vi "HC-Bal_Calc.vi"(7 "Omicron?":bool, 8 "HC Bal Transient":dbl, 9 "HC Bal Factor":dbl, 10 "Air_Inj":dbl[](array[numeric]), 11 "Air_Bal_Array":dbl[](array[numeric])) -> (2 "HC Bal Inj":dbl)   [LabVIEW 2014]
panel:
  # "HC Balance Calculation"
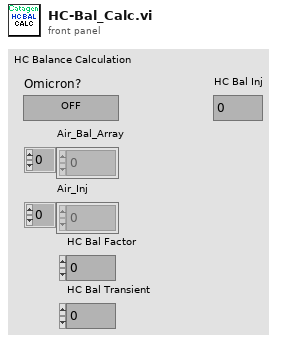
[diagram p1: front panel]
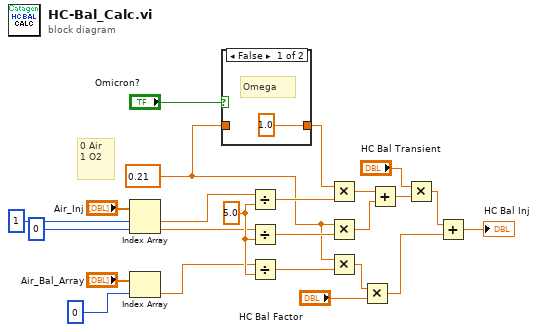
[diagram p0: block diagram]
diagram:
  w2 = 0.21 ("x")
  w22 = 5.0 ("y")
  # "0 Air\n1 O2"
  n1 = Index Array(array="Air_Inj", index #1=1 ("index"), index #2=0 ("index")) -> (element #1=w18:dbl, element #2=w17:dbl)
  n2 = Index Array(array="Air_Bal_Array", index=0) -> (element=w15:dbl)
  n3 = case shown="False" "Omicron?" {
    tunnel: [1.0 ("x") w26] -> w3
    tunnel: w2 -> [_ w26]
    frame False {
      # "Omega"
    }
    frame True {
      # "Omicron"
    }
  }
  n4 = Divide(x=w18, y=w22) -> (x/y=w21:dbl)
  n5 = Divide(x=w17, y=w22) -> (x/y=w20:dbl)
  n6 = Divide(x=w15, y=w22) -> (x/y=w19:dbl)
  n7 = Multiply(x=w3, y=w21) -> (x*y=w12:dbl)
  n8 = Multiply(x=w2, y=w20) -> (x*y=w11:dbl)
  n9 = Multiply(x=w2, y=w19) -> (x*y=w14:dbl)
  n10 = Multiply(x=w14, y="HC Bal Factor") -> (x*y=w9:dbl)
  n11 = Add(x=w12, y=w11) -> (x+y=w8:dbl)
  n12 = Multiply(x="HC Bal Transient", y=w8) -> (x*y=w7:dbl)
  n13 = Add(x=w7, y=w9) -> (x+y=→"HC Bal Inj":dbl)
